vi "Find_One_Second.vi"(8 "Status/Errors in":refnum<vi>, 9 "Master?":T1, 10 "GPS timestamp in":T2, 11 "One Second in":T3[](array[typedef]) {"Ch1 High" format="%0.0f"}) -> (0 "Status/Errors out":refnum<vi>, 1 "Wait for One Seconds?":bool, 2 "Found One Seconds?":bool, 3 "One Second out":T3[](array[typedef]) {"Ch1 High" format="%0.0f"}, 4 "No 1 sec?":bool)   [LabVIEW 2010]
uses:
  Controls/One_Second.ctl
  Controls/GPS_Timestamp.ctl
  Controls/Master.ctl
  Controls/Add_Subtract.ctl
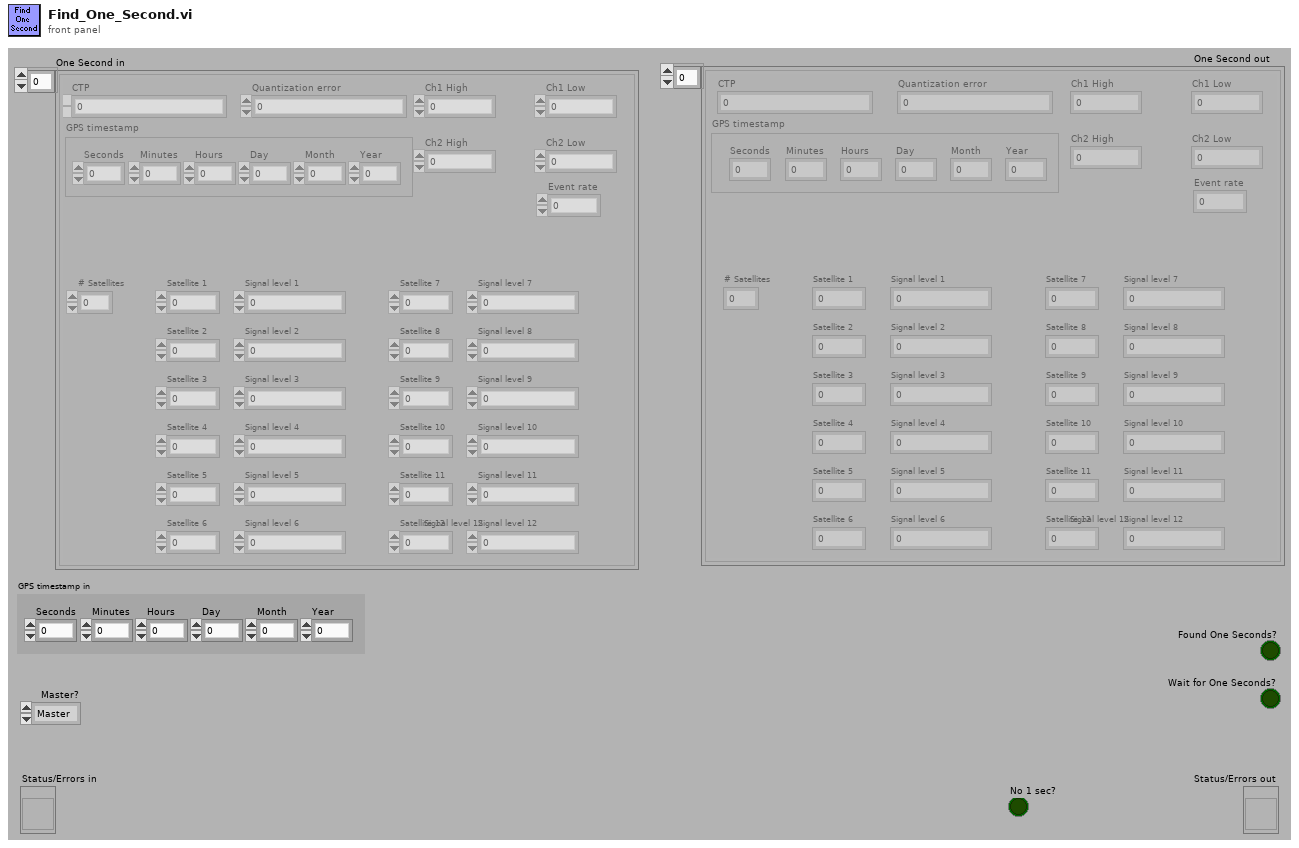
[diagram p1: front panel]
types:
  T1 = typedef "Master.ctl" = enum16{"Master", "Slave", "General"}
  T2 = typedef "GPS_Timestamp.ctl" = cluster{"Seconds":u8, "Minutes":u8, "Hours":u8, "Day":u8, "Month":u8, "Year":u16}
  T3 = typedef "One_Second.ctl" = cluster{"GPS timestamp":T2, "CTP":u32, "Quantization error":u32, "Ch1 High":u16, "Ch1 Low":u16, "Ch2 High":u16, "Ch2 Low":u16, "Event rate":u16, "# Satellites":u8, "Satellite 1":u8, "Satellite 2":u8, "Satellite 3":u8, "Satellite 4":u8, "Satellite 5":u8, "Satellite 6":u8, "Signal level 1":sgl, "Signal level 2":sgl, "Signal level 3":sgl, "Signal level 4":sgl, "Signal level 5":sgl, "Signal level 6":sgl, "Satellite 7":u8, "Satellite 8":u8, "Satellite 9":u8, "Satellite 10":u8, "Satellite 11":u8, "Satellite 12":u8, "Signal level 7":sgl, "Signal level 8":sgl, "Signal level 9":sgl, "Signal level 10":sgl, "Signal level 11":sgl, "Signal level 12":sgl}
  T4 = typedef "Comparison_Result.ctl" = enum16{"equal", "1 < 2", "1 > 2", "error in 1", "error in 2", "error in both"}
  T5 = typedef "Add_Subtract.ctl" = enum16{"Add", "Subtract"}
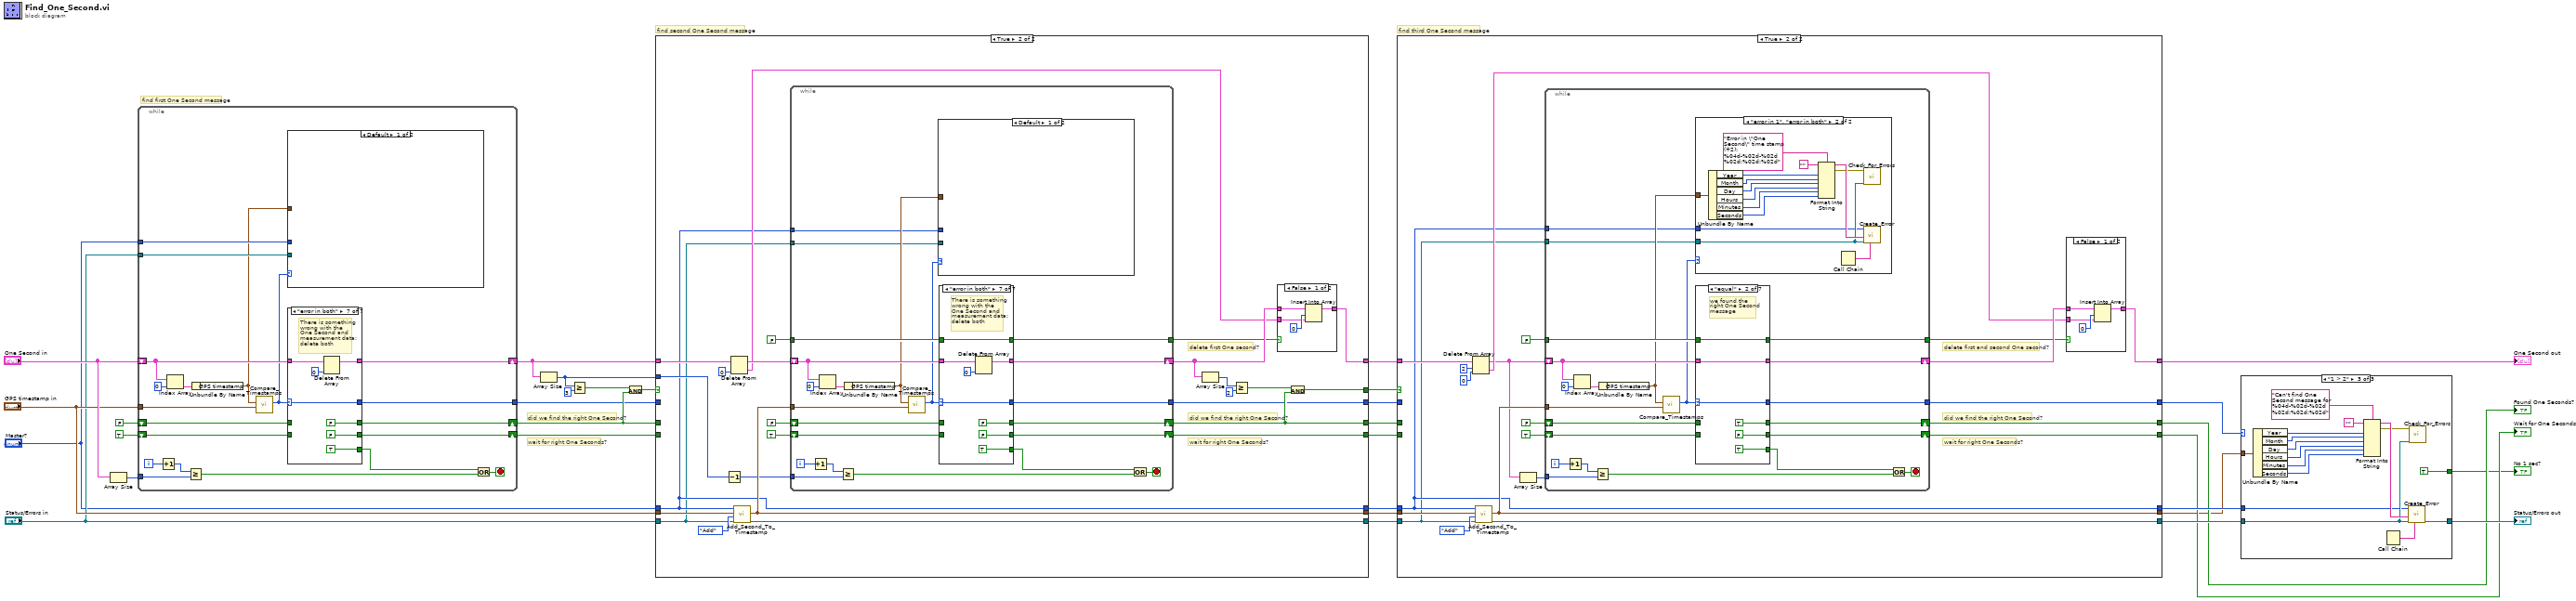
[diagram p0: block diagram]
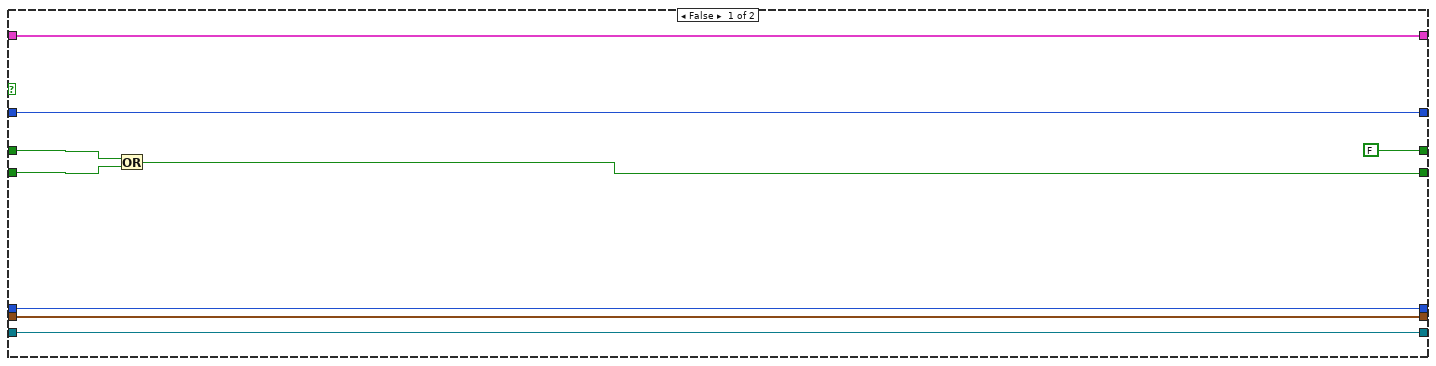
[diagram p2: hidden frame]
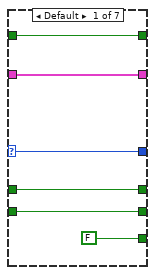
[diagram p5: hidden frame]
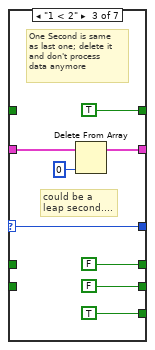
[diagram p6: hidden frame]
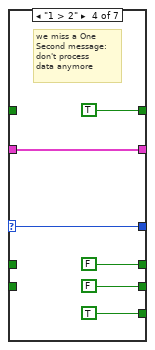
[diagram p7: hidden frame]
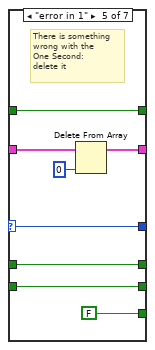
[diagram p8: hidden frame]
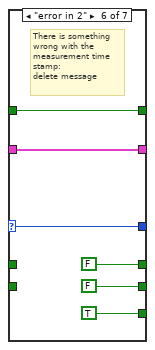
[diagram p9: hidden frame]
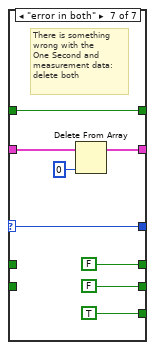
[diagram p10: hidden frame]
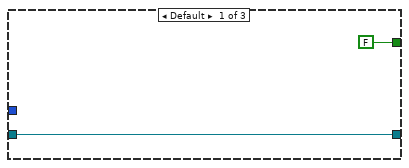
[diagram p11: hidden frame]
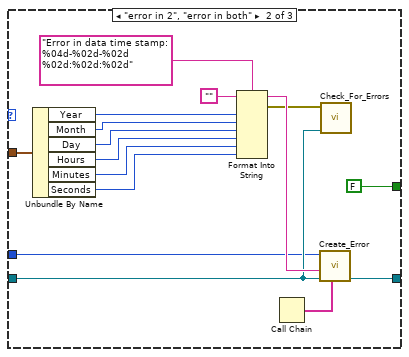
[diagram p12: hidden frame]
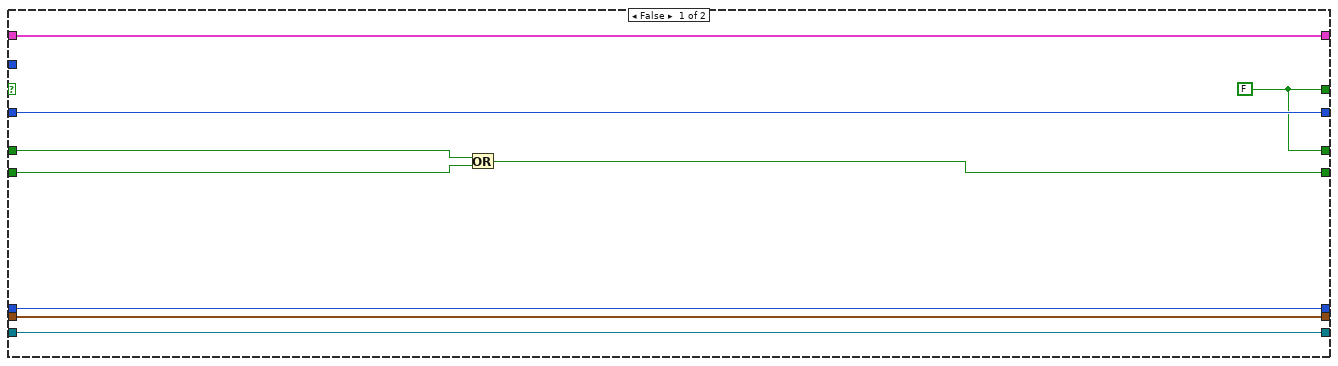
[diagram p13: hidden frame]
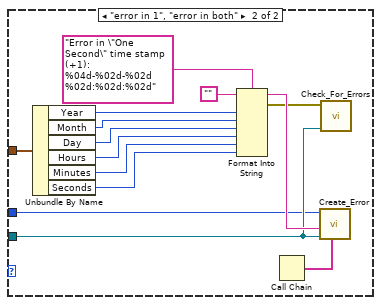
[diagram p15: hidden frame]
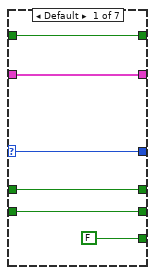
[diagram p16: hidden frame]
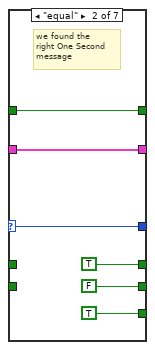
[diagram p17: hidden frame]
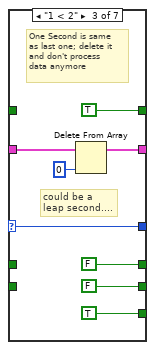
[diagram p18: hidden frame]
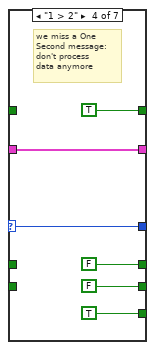
[diagram p19: hidden frame]
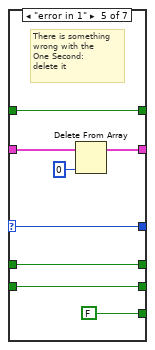
[diagram p20: hidden frame]
diagram:
  # "find third One Second message"
  # "find second One Second message"
  # "find first One Second message"
  # "wait for right One Seconds?"
  # "did we find the right One Second?"
  n1 = Array Size(array="One Second in") -> (size(s)=w29:i32)
  n2 = while {
    tunnel: "GPS timestamp in" -> [w50]
    tunnel: w29 -> [w40]
    shift-right: [w46] -> w26
    shift-left: "One Second in" -> [w47]
    shift-right: [w44] -> w14
    shift-left: TRUE -> [w43]
    shift-right: [w49] -> w13
    shift-left: FALSE -> [w42]
    tunnel: [w37] -> w7
    tunnel: "Status/Errors in" -> [w36]
    tunnel: "Master?" -> [w35]
    i -> [w41]
    stop <- w51 stop-if-true
    n3 = Increment(x=w41) -> (x+1=w39:i32)
    n4 = Index Array(array=w47, index=0) -> (element=w52:T3)
    n5 = Greater Or Equal?(x=w39, y=w40) -> (x >= y?=w38:bool)
    n6 = Unbundle By Name(w52) -> ("GPS timestamp"=w33:T2)
    n7 = call "Compare_Timestamps.vi"("Time stamp 2"=w50, "Time stamp 1"=w33) -> ("Comparison result"=w34:T4)  [unwired: 9 out]
    n8 = case shown="Default" w34 {
      tunnel: w36 -> [_ w55]
      tunnel: w33 -> [_ w65]
      tunnel: w35 -> [_ w53]
      frame Default {
      }
      frame "error in 1", "error in both" {
        n9 = Unbundle By Name(w65) -> ("Year"=w62:u16, "Month"=w61:u8, "Day"=w60:u8, "Hours"=w59:u8, "Minutes"=w58:u8, "Seconds"=w57:u8)
        n10 = Format Into String(format string="Error in \"One Second\" time stamp: %04d-%02d-%02d %02d:%02d:%02d", initial string="", w62, w61, w60, w59, w58, w57) -> (resulting string=w56:string, error out=w54:errorcluster)  [unwired: 1 in]
        n11 = Call Chain() -> (call chain=w66:string[])
        n12 = call "Create_Error.vi"("Call chain"=w66, "Status/Errors in"=w55, "HiSPARC error"=w56, "Master?"=w53) -> ()  [unwired: 2 in, 6 out]
        n13 = call "Check_For_Errors.vi"("Status/Errors in"=w55, "error in"=w54) -> ()  [unwired: 10 out]
      }
    }
    n14 = case shown="\"error in both\"" w34 {
      selector: w34 -> [w67 w73 w77 w84 w89 w96 w104]
      tunnel: [w69 TRUE w78 FALSE w90 FALSE FALSE] -> w49
      tunnel: [FALSE TRUE FALSE TRUE FALSE TRUE TRUE] -> w48
      tunnel: w47 -> [w71 w75 w83 w88 w92 w100 w105]
      tunnel: [w71 w75 w81 w88 w93 w100 w106] -> w46
      tunnel: [w70 FALSE w79 FALSE w91 FALSE FALSE] -> w44
      tunnel: w43 -> [w70 _ w79 _ w91 _ _]
      tunnel: w42 -> [w69 _ w78 _ w90 _ _]
      tunnel: [w67 w73 w77 w84 w89 w96 w104] -> w37
      frame Default {
      }
      frame "equal" {
        # "we found the\nright One Second\nmessage"
      }
      frame "1 < 2" {
        # "One Second is\nold; delete it"
        n15 = Delete From Array(array=w83, index=0) -> (array with subset deleted=w81:T3[])  [unwired: 1 in, 1 out]
      }
      frame "1 > 2" {
        # "message is old;\nwe can't process it"
      }
      frame "error in 1" {
        # "There is something\nwrong with the\nOne Second:\ndelete it"
        n16 = Delete From Array(array=w92, index=0) -> (array with subset deleted=w93:T3[])  [unwired: 1 in, 1 out]
      }
      frame "error in 2" {
        # "There is something\nwrong with the\nmeasurement time\nstamp:\ndelete message"
      }
      frame "error in both" {
        # "There is something\nwrong with the\nOne Second and\nmeasurement data:\ndelete both"
        n17 = Delete From Array(array=w105, index=0) -> (array with subset deleted=w106:T3[])  [unwired: 1 in, 1 out]
      }
    }
    n18 = Or(x=w48, y=w38) -> (x .or. y?=w51:bool)
  }
  n19 = Array Size(array=w26) -> (size(s)=w4:i32)
  n20 = Greater Or Equal?(x=w4, y=3) -> (x >= y?=w24:bool)
  n21 = And(x=w24, y=w13) -> (x .and. y?=w23:bool)
  n22 = case shown="True" w23 {
    tunnel: "GPS timestamp in" -> [w114 w141]
    tunnel: "Master?" -> [w113 w118]
    tunnel: "Status/Errors in" -> [w115 w117]
    tunnel: [w115 w140] -> w20
    tunnel: w26 -> [w116 w131]
    tunnel: w4 -> [_ w120]
    tunnel: [w111 w133] -> w21
    tunnel: [w116 w125] -> w22
    tunnel: [w114 w124] -> w19
    tunnel: [w113 w118] -> w18
    tunnel: w14 -> [w109 _]
    tunnel: w13 -> [w110 _]
    tunnel: [w111 w122] -> w12
    tunnel: [w108 w123] -> w11
    tunnel: w7 -> [w112 _]
    tunnel: [w112 w121] -> w6
    frame False {
      w111 = FALSE
      n23 = Or(x=w110, y=w109) -> (x .or. y?=w108:bool)
    }
    frame True {
      # "delete first One second?"
      # "wait for right One Seconds?"
      # "did we find the right One Second?"
      n24 = Decrement(x=w120) -> (x-1=w119:i32)
      n25 = Delete From Array(array=w131, index=0) -> (deleted portion=w127:T3, array with subset deleted=w130:T3[])  [unwired: 1 in]
      n26 = call "Add_Second_To_Timestamp.vi"("Status/Errors in"=w117, "Add/Subtract"=Add_Subtract."Add", "Time stamp"=w141, "Master?"=w118) -> ("Status/Errors out"=w140:refnum<vi>, "Time stamp out"=w124:T2)  [unwired: 6 out]
      n27 = while {
        tunnel: w124 -> [w166]
        tunnel: w119 -> [w155]
        shift-right: [w162] -> w128
        shift-left: w130 -> [w163]
        shift-right: [w160] -> w123
        shift-left: TRUE -> [w159]
        shift-right: [w165] -> w122
        shift-left: FALSE -> [w158]
        tunnel: [w157] -> w121
        tunnel: [w152] -> w126
        tunnel: FALSE -> [w151]
        tunnel: w118 -> [w147]
        tunnel: w117 -> [w148]
        i -> [w156]
        stop <- w167 stop-if-true
        n28 = Increment(x=w156) -> (x+1=w154:i32)
        n29 = Index Array(array=w163, index=0) -> (element=w168:T3)
        n30 = Greater Or Equal?(x=w154, y=w155) -> (x >= y?=w153:bool)
        n31 = Unbundle By Name(w168) -> ("GPS timestamp"=w150:T2)
        n32 = call "Compare_Timestamps.vi"("Time stamp 2"=w166, "Time stamp 1"=w150) -> ("Comparison result"=w149:T4)  [unwired: 9 out]
        n33 = case shown="Default" w149 {
          tunnel: w148 -> [_ w172]
          tunnel: w150 -> [_ w181]
          tunnel: w147 -> [_ w170]
          frame Default {
          }
          frame "error in 1", "error in both" {
            n34 = Unbundle By Name(w181) -> ("Year"=w179:u16, "Month"=w178:u8, "Day"=w177:u8, "Hours"=w176:u8, "Minutes"=w175:u8, "Seconds"=w174:u8)
            n35 = Format Into String(format string="Error in \"One Second\" time stamp (+1): %04d-%02d-%02d %02d:%02d:%02d", initial string="", w179, w178, w177, w176, w175, w174) -> (resulting string=w173:string, error out=w171:errorcluster)  [unwired: 1 in]
            n36 = Call Chain() -> (call chain=w182:string[])
            n37 = call "Create_Error.vi"("Call chain"=w182, "Status/Errors in"=w172, "HiSPARC error"=w173, "Master?"=w170) -> ()  [unwired: 2 in, 6 out]
            n38 = call "Check_For_Errors.vi"("Status/Errors in"=w172, "error in"=w171) -> ()  [unwired: 10 out]
          }
        }
        n39 = case shown="\"error in both\"" w149 {
          selector: w149 -> [w184 w191 w198 w204 w210 w218 w227]
          tunnel: [w186 TRUE FALSE FALSE w211 FALSE FALSE] -> w165
          tunnel: [FALSE TRUE TRUE TRUE FALSE TRUE TRUE] -> w164
          tunnel: w163 -> [w188 w193 w202 w208 w213 w222 w229]
          tunnel: [w188 w193 w200 w208 w214 w222 w228] -> w162
          tunnel: [w187 FALSE FALSE FALSE w212 FALSE FALSE] -> w160
          tunnel: w159 -> [w187 _ _ _ w212 _ _]
          tunnel: w158 -> [w186 _ _ _ w211 _ _]
          tunnel: [w184 w191 w198 w204 w210 w218 w227] -> w157
          tunnel: [w183 w189 TRUE TRUE w209 w217 w223] -> w152
          tunnel: w151 -> [w183 w189 _ _ w209 w217 w223]
          frame Default {
          }
          frame "equal" {
            # "we found the\nright One Second\nmessage"
          }
          frame "1 < 2" {
            # "could be a\nleap second...."
            # "One Second is same\nas last one; delete it\nand don't process\ndata anymore"
            n40 = Delete From Array(array=w202, index=0) -> (array with subset deleted=w200:T3[])  [unwired: 1 in, 1 out]
          }
          frame "1 > 2" {
            # "we miss a One\nSecond message:\ndon't process\ndata anymore"
          }
          frame "error in 1" {
            # "There is something\nwrong with the\nOne Second:\ndelete it"
            n41 = Delete From Array(array=w213, index=0) -> (array with subset deleted=w214:T3[])  [unwired: 1 in, 1 out]
          }
          frame "error in 2" {
            # "There is something\nwrong with the\nmeasurement time\nstamp:\ndelete message"
          }
          frame "error in both" {
            # "There is something\nwrong with the\nOne Second and\nmeasurement data:\ndelete both"
            n42 = Delete From Array(array=w229, index=0) -> (array with subset deleted=w228:T3[])  [unwired: 1 in, 1 out]
          }
        }
        n43 = Or(x=w164, y=w153) -> (x .or. y?=w167:bool)
      }
      n44 = Array Size(array=w128) -> (size(s)=w134:i32)
      n45 = Greater Or Equal?(x=w134, y=2) -> (x >= y?=w135:bool)
      n46 = case shown="False" w126 {
        tunnel: w128 -> [w144 w146]
        tunnel: w127 -> [w143 _]
        tunnel: [w142 w146] -> w125
        frame False {
          n47 = Insert Into Array(array=w144, index=0, new element=w143) -> (w142:T3[])
        }
        frame True {
        }
      }
      n48 = And(x=w135, y=w122) -> (x .and. y?=w133:bool)
    }
  }
  n49 = case shown="True" w21 {
    tunnel: w19 -> [w236 w260]
    tunnel: w18 -> [w237 w241]
    tunnel: w20 -> [w238 w240]
    tunnel: [w238 w259] -> w16
    tunnel: w22 -> [w239 w254]
    tunnel: [w239 w249] -> w17
    tunnel: [w237 w241] -> w15
    tunnel: w12 -> [w234 _]
    tunnel: w11 -> [w233 _]
    tunnel: [FALSE w246] -> w10
    tunnel: [w232 w247] -> w9
    tunnel: [w236 w245] -> w8
    tunnel: w6 -> [w235 _]
    tunnel: [w235 w244] -> w5
    frame False {
      n50 = Or(x=w234, y=w233) -> (x .or. y?=w232:bool)
    }
    frame True {
      # "delete first and second One second?"
      # "wait for right One Seconds?"
      # "did we find the right One Second?"
      n51 = Delete From Array(array=w254, length=2, index=0) -> (deleted portion=w251:T3[], array with subset deleted=w242:T3[])
      n52 = call "Add_Second_To_Timestamp.vi"("Status/Errors in"=w240, "Add/Subtract"=Add_Subtract."Add", "Time stamp"=w260, "Master?"=w241) -> ("Status/Errors out"=w259:refnum<vi>, "Time stamp out"=w245:T2)  [unwired: 6 out]
      n53 = Array Size(array=w242) -> (size(s)=w243:i32)
      n54 = while {
        tunnel: w245 -> [w285]
        tunnel: w243 -> [w274]
        shift-right: [w281] -> w252
        shift-left: w242 -> [w282]
        shift-right: [w279] -> w247
        shift-left: TRUE -> [w278]
        shift-right: [w284] -> w246
        shift-left: FALSE -> [w277]
        tunnel: [w276] -> w244
        tunnel: [w271] -> w250
        tunnel: FALSE -> [w270]
        tunnel: w241 -> [w268]
        tunnel: w240 -> [w267]
        i -> [w275]
        stop <- w286 stop-if-true
        n55 = Increment(x=w275) -> (x+1=w273:i32)
        n56 = Index Array(array=w282, index=0) -> (element=w287:T3)
        n57 = Greater Or Equal?(x=w273, y=w274) -> (x >= y?=w272:bool)
        n58 = Unbundle By Name(w287) -> ("GPS timestamp"=w269:T2)
        n59 = call "Compare_Timestamps.vi"("Time stamp 2"=w285, "Time stamp 1"=w269) -> ("Comparison result"=w266:T4)  [unwired: 9 out]
        n60 = case shown="\"error in 1\", \"error in both\"" w266 {
          tunnel: w267 -> [_ w291]
          tunnel: w269 -> [_ w300]
          tunnel: w268 -> [_ w289]
          frame Default {
          }
          frame "error in 1", "error in both" {
            n61 = Unbundle By Name(w300) -> ("Year"=w298:u16, "Month"=w297:u8, "Day"=w296:u8, "Hours"=w295:u8, "Minutes"=w294:u8, "Seconds"=w293:u8)
            n62 = Format Into String(format string="Error in \"One Second\" time stamp (+2): %04d-%02d-%02d %02d:%02d:%02d", initial string="", w298, w297, w296, w295, w294, w293) -> (resulting string=w292:string, error out=w290:errorcluster)  [unwired: 1 in]
            n63 = Call Chain() -> (call chain=w301:string[])
            n64 = call "Create_Error.vi"("Call chain"=w301, "Status/Errors in"=w291, "HiSPARC error"=w292, "Master?"=w289) -> ()  [unwired: 2 in, 6 out]
            n65 = call "Check_For_Errors.vi"("Status/Errors in"=w291, "error in"=w290) -> ()  [unwired: 10 out]
          }
        }
        n66 = case shown="\"equal\"" w266 {
          selector: w266 -> [w303 w310 w317 w323 w329 w337 w345]
          tunnel: [w305 TRUE FALSE FALSE w330 FALSE FALSE] -> w284
          tunnel: [FALSE TRUE TRUE TRUE FALSE TRUE TRUE] -> w283
          tunnel: w282 -> [w307 w312 w321 w327 w332 w341 w347]
          tunnel: [w307 w312 w319 w327 w333 w341 w346] -> w281
          tunnel: [w306 FALSE FALSE FALSE w331 FALSE FALSE] -> w279
          tunnel: w278 -> [w306 _ _ _ w331 _ _]
          tunnel: w277 -> [w305 _ _ _ w330 _ _]
          tunnel: [w303 w310 w317 w323 w329 w337 w345] -> w276
          tunnel: [w302 w308 TRUE TRUE w328 w336 w348] -> w271
          tunnel: w270 -> [w302 w308 _ _ w328 w336 w348]
          frame Default {
          }
          frame "equal" {
            # "we found the\nright One Second\nmessage"
          }
          frame "1 < 2" {
            # "could be a\nleap second...."
            # "One Second is same\nas last one; delete it\nand don't process\ndata anymore"
            n67 = Delete From Array(array=w321, index=0) -> (array with subset deleted=w319:T3[])  [unwired: 1 in, 1 out]
          }
          frame "1 > 2" {
            # "we miss a One\nSecond message:\ndon't process\ndata anymore"
          }
          frame "error in 1" {
            # "There is something\nwrong with the\nOne Second:\ndelete it"
            n68 = Delete From Array(array=w332, index=0) -> (array with subset deleted=w333:T3[])  [unwired: 1 in, 1 out]
          }
          frame "error in 2" {
            # "There is something\nwrong with the\nmeasurement time\nstamp:\ndelete message"
          }
          frame "error in both" {
            # "There is something\nwrong with the\nOne Second and\nmeasurement data:\ndelete both"
            n69 = Delete From Array(array=w347, index=0) -> (array with subset deleted=w346:T3[])  [unwired: 1 in, 1 out]
          }
        }
        n70 = Or(x=w283, y=w272) -> (x .or. y?=w286:bool)
      }
      n71 = case shown="False" w250 {
        tunnel: w252 -> [w263 w265]
        tunnel: w251 -> [w261 _]
        tunnel: [w262 w265] -> w249
        frame False {
          n72 = Insert Into Array(array=w263, index=0, new element=w261) -> (w262:T3[])
        }
        frame True {
        }
      }
    }
  }
  "Wait for One Seconds?" <- w9
  "Found One Seconds?" <- w10
  "One Second out" <- w17
  n73 = case shown="\"1 > 2\"" w5 {
    tunnel: [w351 w367 w383] -> w28
    tunnel: w16 -> [w351 w355 w371]
    tunnel: w8 -> [_ w365 w381]
    tunnel: w15 -> [_ w353 w369]
    tunnel: [FALSE FALSE TRUE] -> w1
    frame Default {
    }
    frame "error in 2", "error in both" {
      n74 = Unbundle By Name(w365) -> ("Year"=w362:u16, "Month"=w361:u8, "Day"=w360:u8, "Hours"=w359:u8, "Minutes"=w358:u8, "Seconds"=w357:u8)
      n75 = Format Into String(format string="Error in data time stamp: %04d-%02d-%02d %02d:%02d:%02d", initial string="", w362, w361, w360, w359, w358, w357) -> (resulting string=w356:string, error out=w354:errorcluster)  [unwired: 1 in]
      n76 = Call Chain() -> (call chain=w366:string[])
      n77 = call "Create_Error.vi"("Call chain"=w366, "Status/Errors in"=w355, "HiSPARC error"=w356, "Master?"=w353) -> ("Status/Errors out"=w367:refnum<vi>)  [unwired: 2 in, 5 out]
      n78 = call "Check_For_Errors.vi"("Status/Errors in"=w355, "error in"=w354) -> ()  [unwired: 10 out]
    }
    frame "1 > 2" {
      n79 = Unbundle By Name(w381) -> ("Year"=w378:u16, "Month"=w377:u8, "Day"=w376:u8, "Hours"=w375:u8, "Minutes"=w374:u8, "Seconds"=w373:u8)
      n80 = Format Into String(format string="Can't find One Second message for %04d-%02d-%02d %02d:%02d:%02d", initial string="", w378, w377, w376, w375, w374, w373) -> (resulting string=w372:string, error out=w370:errorcluster)  [unwired: 1 in]
      n81 = Call Chain() -> (call chain=w382:string[])
      n82 = call "Create_Error.vi"("Call chain"=w382, "Status/Errors in"=w371, "HiSPARC error"=w372, "Master?"=w369) -> ("Status/Errors out"=w383:refnum<vi>)  [unwired: 2 in, 5 out]
      n83 = call "Check_For_Errors.vi"("Status/Errors in"=w371, "error in"=w370) -> ()  [unwired: 10 out]
    }
  }
  "Status/Errors out" <- w28
  "No 1 sec?" <- w1
